vi "sensor get num attached dockingstations1.vi"(11 "dest_num_docks":u32) -> (2 "function return":i32, 3 "dest_num_docks out":u32)   [LabVIEW 2019, in "apdm.lvlib"]
doc: "APDM_EXPORT int apdm_sensor_get_num_attached_dockingstations1(uint32_t *dest_num_docks);"
uses:
  apdm.lvlib
  Lee Lab/CP FES Walking 2018/Code/Working/LabVIEW/apdm.dll
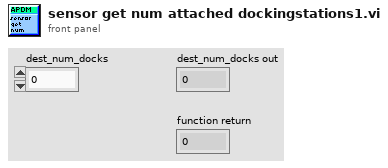
[diagram p1: front panel]
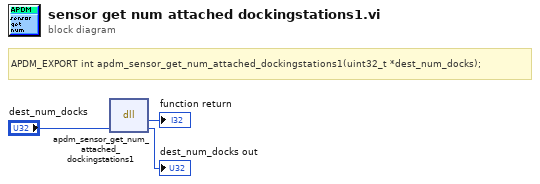
[diagram p0: block diagram]
diagram:
  # "APDM_EXPORT int apdm_sensor_get_num_attached_dockingstations1(uint32_t *dest_num_docks);"
  n1 = dll-call lib="C:/Users/jfalesi/Dropbox/Lee Lab/CP FES Walking 2018/Code/Working/LabVIEW/apdm.*" fn="apdm_sensor_get_num_attached_dockingstations1"("dest_num_docks"="dest_num_docks") -> (→"function return":i32, "dest_num_docks"=→"dest_num_docks out":u32)  [unwired: 3 in, 2 out]
